vi "多功能示波器.vi"(0 "CH1":bool, 1 "frequency":dbl=10.0 caption="频率" min=0.0 max=1000.0 step=1.0, 2 "频率单位":u16(ring) items=["Hz", "KHz"], 3 "amplitude":dbl=1.0 caption="幅值" min=0.0 max=1000.0 step=1.0 format="%0.2p", 4 "幅值单位":u16(ring) items=["V", "mV"], 5 "phase":dbl caption="相位" format="%.2p", 6 "sampling info":cluster{"Fs":dbl, "#s":dbl}={"Fs"=1000.0, "#s"=1000.0} caption="采样信息" {"Fs" format="%.2p"}) -> ()   [LabVIEW 2020]
uses:
  <vilib>/Analysis/4window.llb/windowTd.ctl
  <vilib>/measure/maspectr.llb/Power Spectrum and PSD Export Mode.ctl
  <vilib>/Analysis/3filter.llb/Filter Structure Type.ctl
  <vilib>/measure/maspectr.llb/FFT Power Spectrum and PSD for N Chan.vi
  <vilib>/measure/macond.llb/FIR Filter for N Chan.vi
  <vilib>/measure/macond.llb/IIR Filter for N Chan.vi
  <vilib>/measure/mascope.llb/Cycle Average and RMS 1 chan.vi
  <vilib>/measure/matone.llb/Extract Single Tone Information 1 Chan.vi
  <vilib>/measure/NI_MABase.lvlib
  <vilib>/measure/NI_MAPro.lvlib
  <vilib>/Analysis/NI_AALPro.lvlib
  <vilib>/Analysis/NI_AALBase.lvlib
panel:
  out "波形参数错误":errorcluster
  in  "选项卡控件 3":enum32{"信号发生器 ", " 滤波模式所用的"}(tab)
  in  "开关":bool
  in  "frequency 2":dbl=10.0 caption="频率" min=0.0 max=1000.0 step=1.0
  in  "频率单位 2":u16(ring) items=["Hz", "KHz"]
  in  "amplitude 2":dbl=1.0 caption="幅值" min=0.0 max=1000.0 step=1.0 format="%0.2p"
  in  "幅值单位  2":u16(ring) items=["V", "mV"]
  in  "phase 2":dbl caption="相位" format="%.2p"
  in  "signal type 2":T1(ring) caption="信号类型"
  in  "CH2":bool
  in  "噪音列表 2":u16(ring) items=["无", "高斯噪音", "均匀白噪音"]
  in  "噪音列表":u16(ring) items=["无", "高斯噪音", "均匀白噪音"]
  in  "signal type":T1(ring) caption="信号类型"
  in  "选项卡控件 2":enum32{"FIR滤波器", " IIR滤波器"}(tab)
  in  "FIR filter specifications":T2={"Topology"=enum."Off", "Type"=enum."Lowpass", "#Taps"=50, "Lower PB"=100.0, "Upper PB"=0.0, "Lower SB"=200.0, "Upper SB"=0.0} caption="FIR滤波器规范" {"Lower SB" format="%0.2p"; "Upper SB" format="%0.2p"; "Lower PB" format="%0.2p"; "Upper PB" format="%0.2p"}
  in  "reset filters":bool caption="重置滤波器"
  in  "filter structure option":T3=10 caption="滤波器结构选项" items=["IIR二阶"=0, "IIR四阶"=1, "自动选择"=10]
  in  "reset filter":bool caption="重置滤波器"
  in  "IIR filter specifications":T4={"Topology"=enum."Butterworth", "Type"=enum."Lowpass", "Order"=1, "Lower Fc"=100.0, "Upper Fc"=200.0, "PB Ripple"=1.0, "SB Attenuation"=60.0} caption="IIR滤波器规范" {"PB Ripple" format="%0.2f"; "SB Attenuation" format="%0.2f"; "Lower Fc" format="%0.2p"; "Upper Fc" format="%0.2p"}
  out "错误输出 3":errorcluster caption="滤波器错误输出"
  out "波形保存错误":errorcluster caption="波形保存错误输出"
  in  "选项卡控件":enum32{"示波器", " 功率频谱测量"}(tab)
  in  "滤波模式":bool
  out "字符串 2":string
  out "字符串":string
  in  "停止波形":bool
  in  "波形回放":bool
  in  "波形保存":bool
  in  "V-mV":bool
  in  "Hz-KHz":bool
  in  "幅值 v/div":dbl(knob) scale=0.0..4.0
  in  "时间 s/div":dbl(knob) scale=0.0..5.0
  out "频率":dbl format="%.2p"
  out "周期平均":dbl format="%.2p"
  out "周期均方根":dbl format="%.2p"
  out "相位":dbl format="%.2p"
  out "幅度":dbl format="%.2p"
  out "周期平均 2":dbl caption="周期平均" format="%.2p"
  out "周期均方根 2":dbl caption="周期均方根" format="%.2p"
  out "相位 2":dbl caption="相位" format="%.2p"
  out "幅度 2":dbl caption="幅度" format="%.2p"
  out "频率 2":dbl caption="频率" format="%.2p"
  out "波形图":waveform(dbl)[](graph)
  out "波形图 2":cluster{"f0":dbl, "df":dbl, "magnitude":dbl[]}[](graph)
  in  "averaging parameters":T5={"averaging mode"=enum."No averaging", "weighting mode"=enum."Exponential", "number of averages"=10} caption="平均参数" {"number of averages" min=1}
  out "averaging done":bool caption="完成平均"
  out "averages completed":dbl caption="已完成平均数"
  in  "restart averaging (F)":bool caption="重新开始平均(F)"
  in  "dB On (F)":bool caption="显示为dB(F)"
  in  "window":T6=1 caption="窗" items=["矩形"=0, "Hanning"=1, "Hamming"=2, "Blackman-Harris"=3, "Exact Blackman"=4, "Blackman"=5, "Flat Top"=6, "4阶Blackman-Harris "=7, "7阶Blackman-Harris"=8, "Low Sidelobe"=9, "Blackman Nuttall"=11, "三角"=30, "Bartlett-Hanning"=31, "Bohman"=32, "Parzen"=33, "Welch"=34, "Kaiser"=60, "Dolph-Chebyshev"=61, "高斯"=62]
  in  "window parameter":dbl=nan caption="窗参数"
  in  "export mode":T7 caption="导出模式" items=["功率谱", "功率谱密度"]
  out "error out 2":errorcluster caption="波形保存错误"
  out "error out":errorcluster caption="信号发生错误显示"
  # "信号发生器"
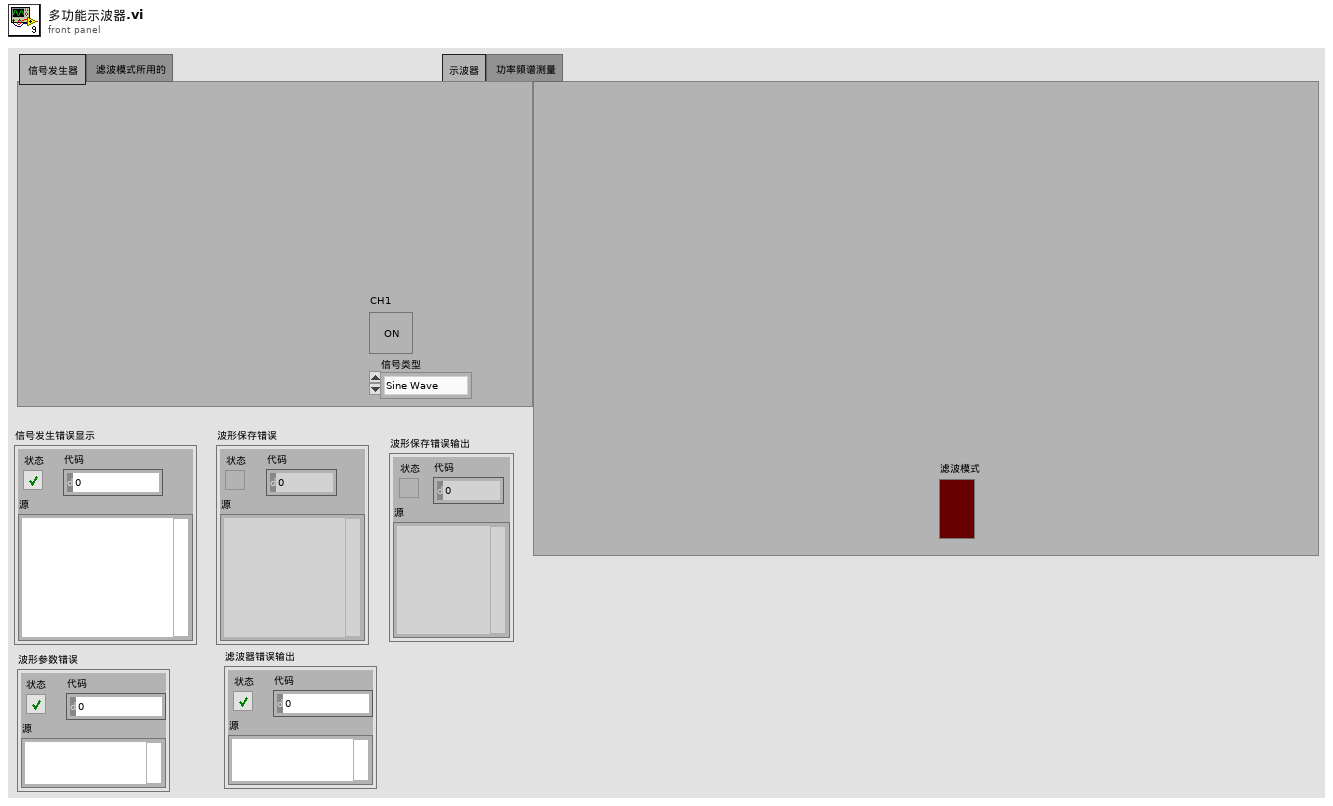
[diagram p1: front panel]
types:
  T1 = enum16{"Sine Wave", "Triangle Wave", "Square Wave", "Sawtooth Wave"}
  T2 = cluster{"Topology":enum16{"Off", "FIR by Specification", "Equi-ripple FIR", "Windowed FIR"}, "Type":enum16{"Lowpass", "Highpass", "Bandpass", "Bandstop"}, "#Taps":i32, "Lower PB":dbl, "Upper PB":dbl, "Lower SB":dbl, "Upper SB":dbl}
  T3 = typedef "NI_AALBase.lvlib/Filter Structure Type.ctl" = u16
  T4 = cluster{"Topology":enum16{"Off", "Butterworth", "Chebyshev", "Inverse Chebyshev", "Elliptic", "Bessel"}, "Type":enum16{"Lowpass", "Highpass", "Bandpass", "Bandstop"}, "Order":i32, "Lower Fc":dbl, "Upper Fc":dbl, "PB Ripple":dbl, "SB Attenuation":dbl}
  T5 = cluster{"averaging mode":enum16{"No averaging", "Vector averaging", "RMS averaging", "Peak hold"}, "weighting mode":enum16{"Linear", "Exponential"}, "number of averages":u32}
  T6 = typedef "NI_AALPro.lvlib/windowTd.ctl" = u32
  T7 = typedef "NI_MAPro.lvlib/Power Spectrum and PSD Export Mode.ctl" = u16
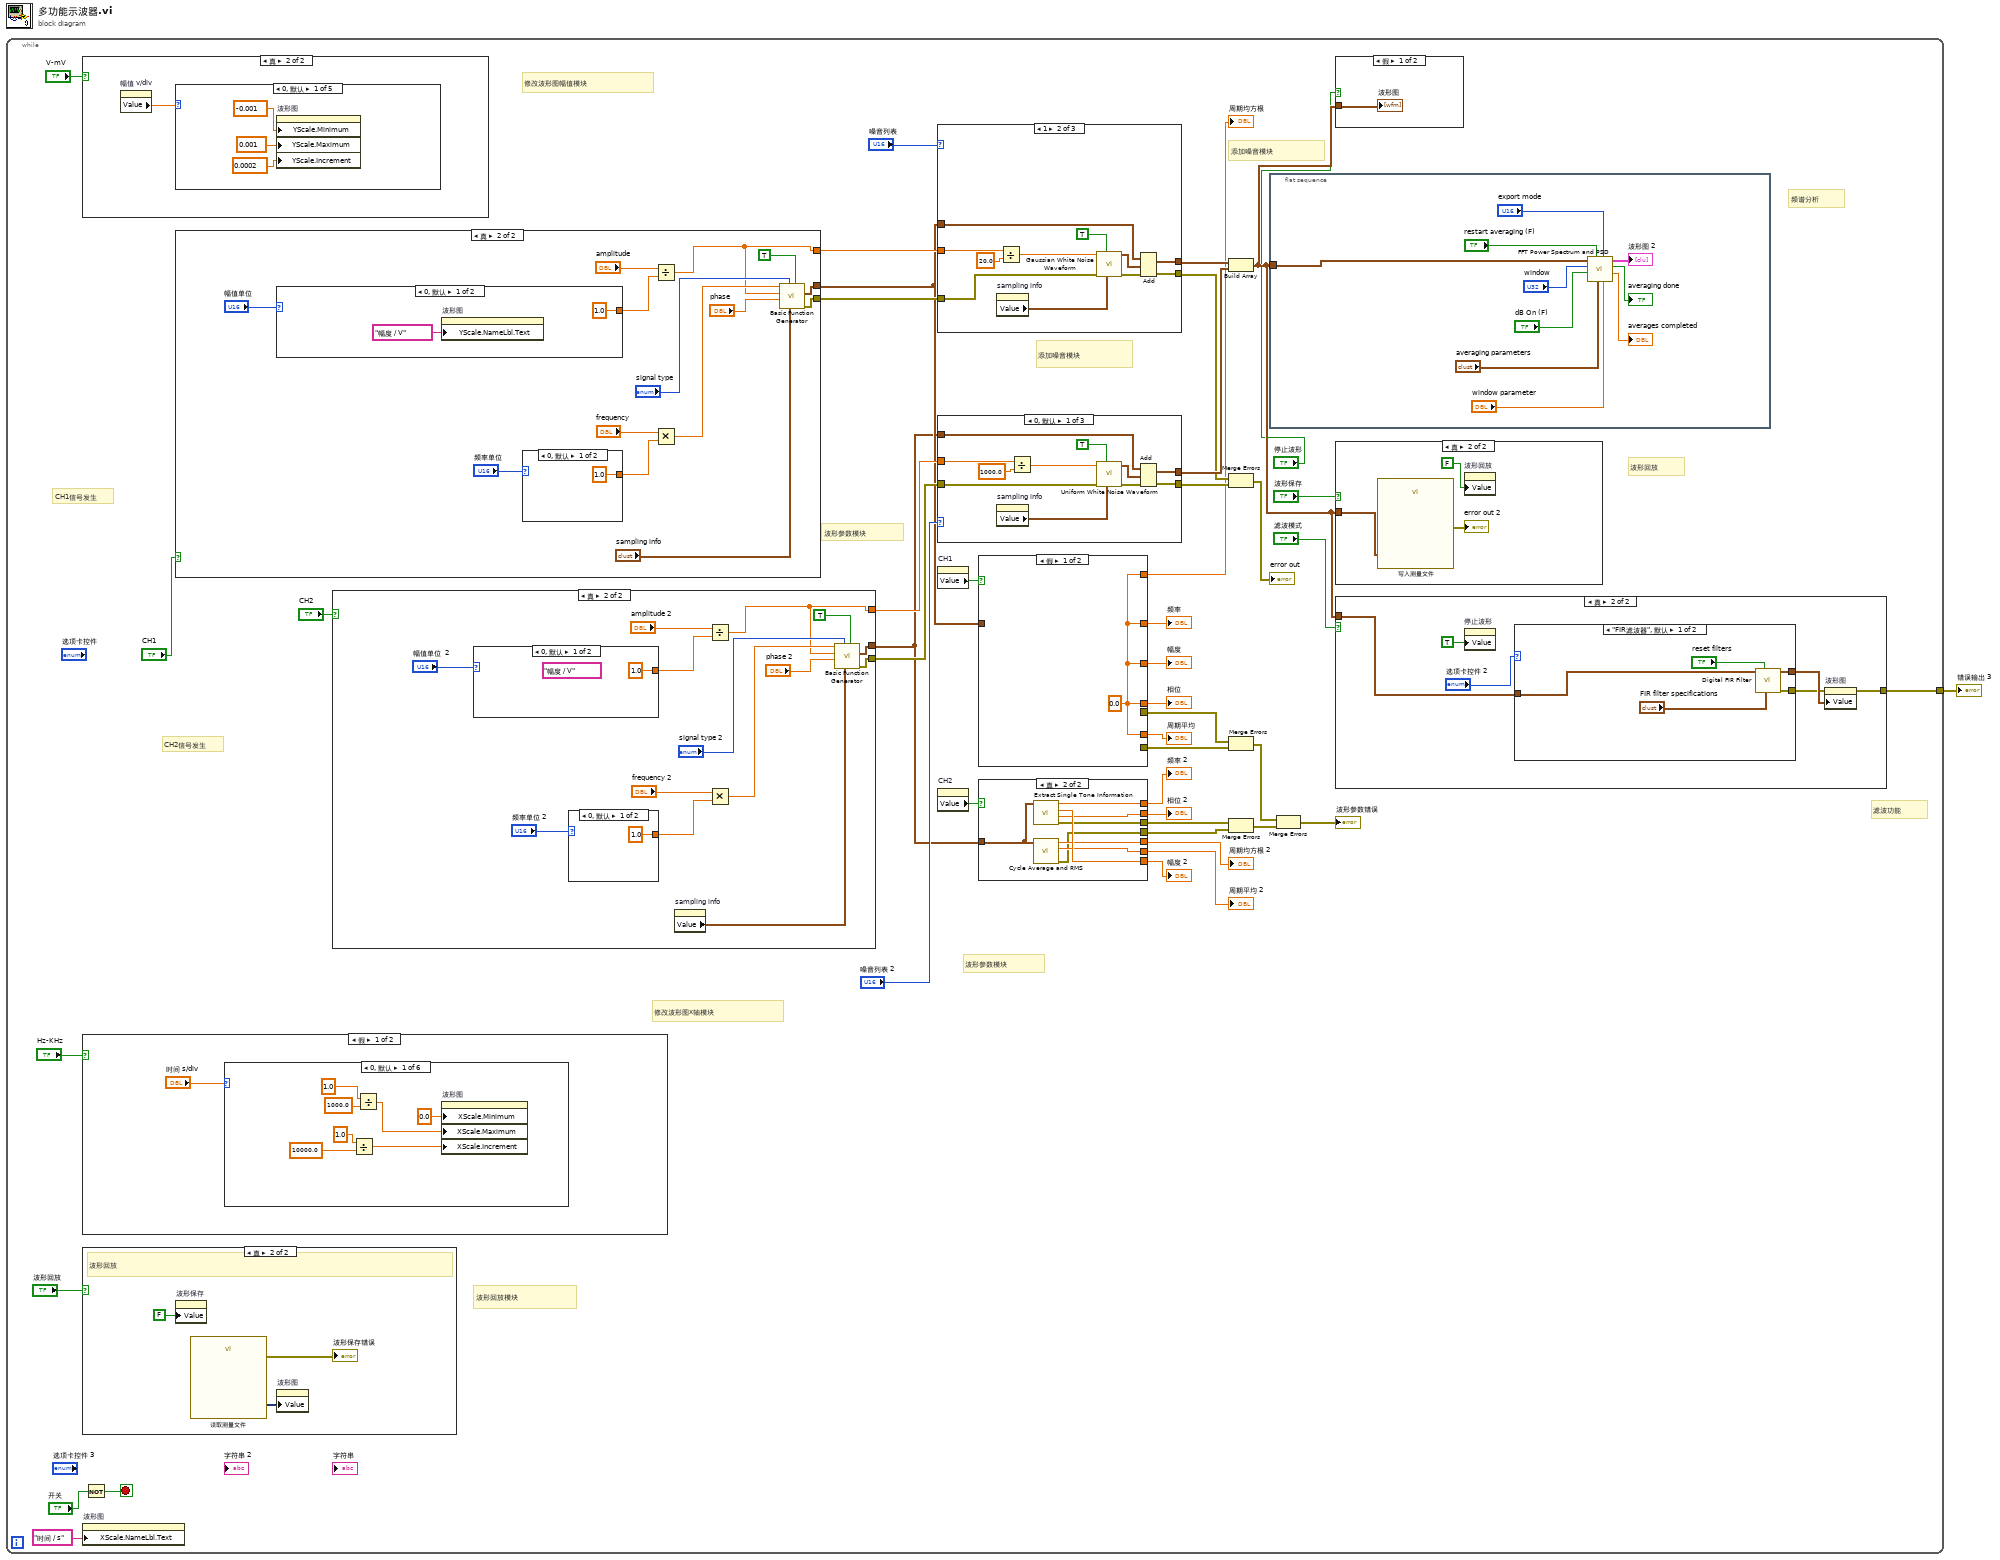
[diagram p0: block diagram]
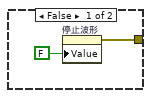
[diagram p2: hidden frame]
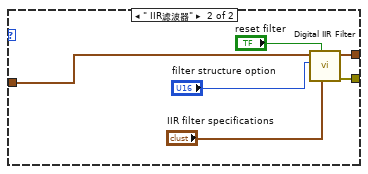
[diagram p3: hidden frame]
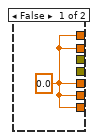
[diagram p4: hidden frame]
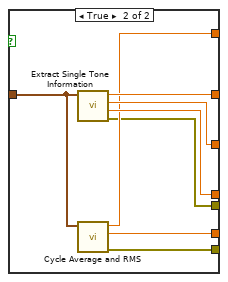
[diagram p5: hidden frame]
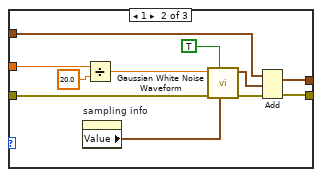
[diagram p9: hidden frame]
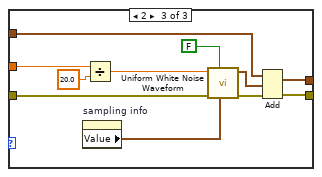
[diagram p10: hidden frame]
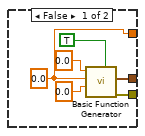
[diagram p11: hidden frame]
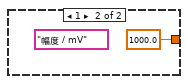
[diagram p12: hidden frame]
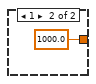
[diagram p13: hidden frame]
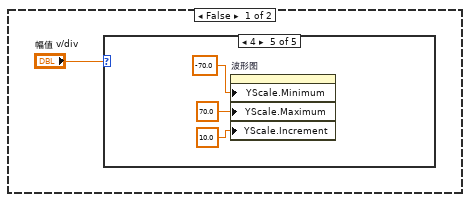
[diagram p14: hidden frame]
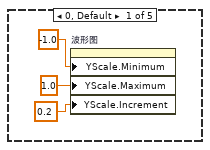
[diagram p15: hidden frame]
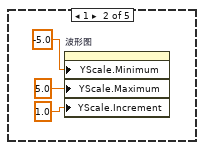
[diagram p16: hidden frame]
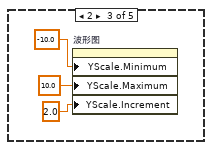
[diagram p17: hidden frame]
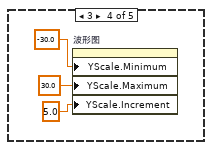
[diagram p18: hidden frame]
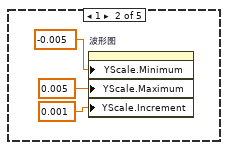
[diagram p19: hidden frame]
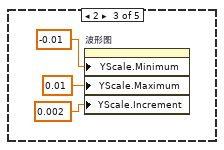
[diagram p20: hidden frame]
diagram:
  n1 = while {
    tunnel: [w5] -> w1
    stop <- w44 stop-if-true
    # "滤波功能"
    # "频谱分析"
    # "波形回放"
    # "波形参数模块"
    # "波形参数模块"
    # "添加噪音模块"
    # "添加噪音模块"
    # "CH2信号发生"
    # "CH1信号发生"
    # "修改波形图x轴模块"
    # "修改波形图幅值模块"
    # "波形回放模块"
    n2 = case shown="真" "V-mV" {
      frame False {
        n3 = case shown="4" "幅值 v/div" {
          frame 0, Default {
            n4 = property on="波形图" class="WFGraph (严格)"("YScale.Minimum"=-1.0 ("Y标尺.范围:最小值"), "YScale.Maximum"=1.0 ("Y标尺.范围:最大值"), "YScale.Increment"=0.2 ("Y标尺.范围:增量")) -> ()  [unwired: 2 in, 2 out]
          }
          frame 1 {
            n5 = property on="波形图" class="WFGraph (严格)"("YScale.Minimum"=-5.0 ("Y标尺.范围:最小值"), "YScale.Maximum"=5.0 ("Y标尺.范围:最大值"), "YScale.Increment"=1.0 ("Y标尺.范围:增量")) -> ()  [unwired: 2 in, 2 out]
          }
          frame 2 {
            n6 = property on="波形图" class="WFGraph (严格)"("YScale.Minimum"=-10.0 ("Y标尺.范围:最小值"), "YScale.Maximum"=10.0 ("Y标尺.范围:最大值"), "YScale.Increment"=2.0 ("Y标尺.范围:增量")) -> ()  [unwired: 2 in, 2 out]
          }
          frame 3 {
            n7 = property on="波形图" class="WFGraph (严格)"("YScale.Minimum"=-30.0 ("Y标尺.范围:最小值"), "YScale.Maximum"=30.0 ("Y标尺.范围:最大值"), "YScale.Increment"=5.0 ("Y标尺.范围:增量")) -> ()  [unwired: 2 in, 2 out]
          }
          frame 4 {
            n8 = property on="波形图" class="WFGraph (严格)"("YScale.Minimum"=-70.0 ("Y标尺.范围:最小值"), "YScale.Maximum"=70.0 ("Y标尺.范围:最大值"), "YScale.Increment"=10.0 ("Y标尺.范围:增量")) -> ()  [unwired: 2 in, 2 out]
          }
        }
      }
      frame True {
        n9 = property on="幅值 v/div" class="Knob (严格)"() -> ("Value"=w174:dbl)  [unwired: 2 in, 2 out]
        n10 = case shown="0, 默认" w174 {
          frame 0, Default {
            n11 = property on="波形图" class="WFGraph (严格)"("YScale.Minimum"=-0.001 ("Y标尺.范围:最小值"), "YScale.Maximum"=0.001 ("Y标尺.范围:最大值"), "YScale.Increment"=0.0002 ("Y标尺.范围:增量")) -> ()  [unwired: 2 in, 2 out]
          }
          frame 1 {
            n12 = property on="波形图" class="WFGraph (严格)"("YScale.Minimum"=-0.005 ("Y标尺.范围:最小值"), "YScale.Maximum"=0.005 ("Y标尺.范围:最大值"), "YScale.Increment"=0.001 ("Y标尺.范围:增量")) -> ()  [unwired: 2 in, 2 out]
          }
          frame 2 {
            n13 = property on="波形图" class="WFGraph (严格)"("YScale.Minimum"=-0.01 ("Y标尺.范围:最小值"), "YScale.Maximum"=0.01 ("Y标尺.范围:最大值"), "YScale.Increment"=0.002 ("Y标尺.范围:增量")) -> ()  [unwired: 2 in, 2 out]
          }
          frame 3 {
            n14 = property on="波形图" class="WFGraph (严格)"("YScale.Minimum"=-0.03 ("Y标尺.范围:最小值"), "YScale.Maximum"=0.03 ("Y标尺.范围:最大值"), "YScale.Increment"=0.005 ("Y标尺.范围:增量")) -> ()  [unwired: 2 in, 2 out]
          }
          frame 4 {
            n15 = property on="波形图" class="WFGraph (严格)"("YScale.Minimum"=-0.07 ("Y标尺.范围:最小值"), "YScale.Maximum"=0.07 ("Y标尺.范围:最大值"), "YScale.Increment"=0.01 ("Y标尺.范围:增量")) -> ()  [unwired: 2 in, 2 out]
          }
        }
      }
    }
    n16 = case shown="假" "Hz-KHz" {
      frame False {
        n17 = case shown="0, 默认" "时间 s/div" {
          frame 0, Default {
            n18 = Divide(x=1.0, y=10000.0) -> (x/y=w191:dbl)
            n19 = Divide(x=1.0, y=1000.0) -> (x/y=w194:dbl)
            n20 = property on="波形图" class="WFGraph (严格)"("XScale.Minimum"=0.0 ("X标尺.范围:最小值"), "XScale.Maximum"=w194, "XScale.Increment"=w191) -> ()  [unwired: 2 in, 2 out]
          }
          frame 1 {
            n21 = Divide(x=1.0, y=1000.0) -> (x/y=w198:dbl)
            n22 = Divide(x=1.0, y=100.0) -> (x/y=w201:dbl)
            n23 = property on="波形图" class="WFGraph (严格)"("XScale.Minimum"=0.0 ("X标尺.范围:最小值"), "XScale.Maximum"=w201, "XScale.Increment"=w198) -> ()  [unwired: 2 in, 2 out]
          }
          frame 2 {
            n24 = Divide(x=5.0, y=1000.0) -> (x/y=w205:dbl)
            n25 = Divide(x=5.0, y=100.0) -> (x/y=w208:dbl)
            n26 = property on="波形图" class="WFGraph (严格)"("XScale.Minimum"=0.0 ("X标尺.范围:最小值"), "XScale.Maximum"=w208, "XScale.Increment"=w205) -> ()  [unwired: 2 in, 2 out]
          }
          frame 3 {
            n27 = Divide(x=1.0, y=10.0) -> (x/y=w215:dbl)
            n28 = Divide(x=1.0, y=100.0) -> (x/y=w212:dbl)
            n29 = property on="波形图" class="WFGraph (严格)"("XScale.Minimum"=0.0 ("X标尺.范围:最小值"), "XScale.Maximum"=w215, "XScale.Increment"=w212) -> ()  [unwired: 2 in, 2 out]
          }
          frame 4 {
            n30 = Divide(x=15.0, y=1000.0) -> (x/y=w219:dbl)
            n31 = Divide(x=15.0, y=100.0) -> (x/y=w222:dbl)
            n32 = property on="波形图" class="WFGraph (严格)"("XScale.Minimum"=0.0 ("X标尺.范围:最小值"), "XScale.Maximum"=w222, "XScale.Increment"=w219) -> ()  [unwired: 2 in, 2 out]
          }
          frame 5 {
            n33 = Divide(x=2.0, y=10.0) -> (x/y=w232:dbl)
            n34 = Divide(x=2.0, y=100.0) -> (x/y=w231:dbl)
            n35 = property on="波形图" class="WFGraph (严格)"("XScale.Minimum"=0.0 ("X标尺.范围:最小值"), "XScale.Maximum"=w232, "XScale.Increment"=w231) -> ()  [unwired: 2 in, 2 out]
          }
        }
      }
      frame True {
        n36 = property on="时间 s/div" class="Knob (严格)"() -> ("Value"=w233:dbl)  [unwired: 2 in, 2 out]
        n37 = case shown="4" w233 {
          frame 0, Default {
            n38 = Divide(x=1.0, y=1000000.0) -> (x/y=w237:dbl)
            n39 = Divide(x=1.0, y=10000000.0) -> (x/y=w234:dbl)
            n40 = property on="波形图" class="WFGraph (严格)"("XScale.Minimum"=0.0 ("X标尺.范围:最小值"), "XScale.Maximum"=w237, "XScale.Increment"=w234) -> ()  [unwired: 2 in, 2 out]
          }
          frame 1 {
            n41 = Divide(x=1.0, y=100000.0) -> (x/y=w244:dbl)
            n42 = Divide(x=1.0, y=1000000.0) -> (x/y=w241:dbl)
            n43 = property on="波形图" class="WFGraph (严格)"("XScale.Minimum"=0.0 ("X标尺.范围:最小值"), "XScale.Maximum"=w244, "XScale.Increment"=w241) -> ()  [unwired: 2 in, 2 out]
          }
          frame 2 {
            n44 = Divide(x=5.0, y=100000.0) -> (x/y=w251:dbl)
            n45 = Divide(x=5.0, y=1000000.0) -> (x/y=w248:dbl)
            n46 = property on="波形图" class="WFGraph (严格)"("XScale.Minimum"=0.0 ("X标尺.范围:最小值"), "XScale.Maximum"=w251, "XScale.Increment"=w248) -> ()  [unwired: 2 in, 2 out]
          }
          frame 3 {
            n47 = Divide(x=1.0, y=10000.0) -> (x/y=w258:dbl)
            n48 = Divide(x=1.0, y=100000.0) -> (x/y=w255:dbl)
            n49 = property on="波形图" class="WFGraph (严格)"("XScale.Minimum"=0.0 ("X标尺.范围:最小值"), "XScale.Maximum"=w258, "XScale.Increment"=w255) -> ()  [unwired: 2 in, 2 out]
          }
          frame 4 {
            n50 = Divide(x=15.0, y=100000.0) -> (x/y=w265:dbl)
            n51 = Divide(x=15.0, y=1000000.0) -> (x/y=w262:dbl)
            n52 = property on="波形图" class="WFGraph (严格)"("XScale.Minimum"=0.0 ("X标尺.范围:最小值"), "XScale.Maximum"=w265, "XScale.Increment"=w262) -> ()  [unwired: 2 in, 2 out]
          }
          frame 5 {
            n53 = Divide(x=2.0, y=10000.0) -> (x/y=w275:dbl)
            n54 = Divide(x=2.0, y=100000.0) -> (x/y=w274:dbl)
            n55 = property on="波形图" class="WFGraph (严格)"("XScale.Minimum"=0.0 ("X标尺.范围:最小值"), "XScale.Maximum"=w275, "XScale.Increment"=w274) -> ()  [unwired: 2 in, 2 out]
          }
        }
      }
    }
    n56 = case shown="真" "波形回放" {
      frame False {
      }
      frame True {
        # "波形回放"
        n57 = property on="波形保存" class="Bool (严格)"("Value"=FALSE ("波形保存")) -> ()  [unwired: 2 in, 2 out]
        n58 = call "读取测量文件"() -> ("error out"=→"波形保存错误":errorcluster, "Signals"=w97:dynamicdata)  [unwired: 6 in, 4 out]
        n59 = property on="波形图" class="WFGraph (严格)"("Value"=w97) -> ()  [unwired: 2 in, 2 out]
      }
    }
    n60 = property on="波形图" class="WFGraph (严格)"("XScale.NameLbl.Text"="时间 / s" ("X标尺.名称标签.文本")) -> ()  [unwired: 2 in, 2 out]
    n61 = Not(x="开关") -> (.not. x?=w44:bool)
    n62 = case shown="真" "CH1" {
      tunnel: [w312 w318] -> w26
      tunnel: [w311 w317] -> w42
      tunnel: [w310 w316] -> w41
      frame False {
        w310 = 0.0 ("amplitude")
        n63 = property on="sampling info" class="Clust (严格)"() -> ("Value"=w309:cluster{"Fs":dbl, "#s":dbl})  [unwired: 2 in, 2 out]
        n64 = call <vilib>:"Basic Function Generator.vi"("reset signal"=TRUE, "sampling info"=w309, "phase"=0.0, "amplitude"=w310, "frequency"=0.0) -> ("error out"=w311:errorcluster, "signal out"=w312:waveform(dbl))  [unwired: 4 in, 1 out]
      }
      frame True {
        n65 = case shown="0, 默认" "幅值单位" {
          tunnel: [1.0 1000.0] -> w322
          frame 0, Default {
            n66 = property on="波形图" class="WFGraph (严格)"("YScale.NameLbl.Text"="幅度 / V") -> ()  [unwired: 2 in, 2 out]
          }
          frame 1 {
            n67 = property on="波形图" class="WFGraph (严格)"("YScale.NameLbl.Text"="幅度 / mV") -> ()  [unwired: 2 in, 2 out]
          }
        }
        n68 = case shown="0, 默认" "频率单位" {
          tunnel: [1.0 1000.0] -> w327
          frame 0, Default {
          }
          frame 1 {
          }
        }
        n69 = Divide(x="amplitude", y=w322) -> (x/y=w316:dbl)
        n70 = Multiply(x="frequency", y=w327) -> (x*y=w326:dbl)
        n71 = call <vilib>:"Basic Function Generator.vi"("reset signal"=TRUE, "sampling info"="sampling info", "signal type"="signal type", "phase"="phase", "amplitude"=w316, "frequency"=w326) -> ("error out"=w317:errorcluster, "signal out"=w318:waveform(dbl))  [unwired: 3 in, 1 out]
      }
    }
    n72 = case shown="真" "CH2" {
      tunnel: [w136 w143] -> w10
      tunnel: [w135 w142] -> w36
      tunnel: [w134 w141] -> w37
      frame False {
        w134 = 0.0 ("amplitude")
        n73 = call <vilib>:"Basic Function Generator.vi"("reset signal"=TRUE, "phase"=0.0, "amplitude"=w134, "frequency"=0.0) -> ("error out"=w135:errorcluster, "signal out"=w136:waveform(dbl))  [unwired: 5 in, 1 out]
      }
      frame True {
        n74 = case shown="0, 默认" "幅值单位  2" {
          tunnel: [1.0 1000.0] -> w147
          frame 0, Default {
            (unwired) "幅度 / V"
          }
          frame 1 {
            (unwired) "幅度 / mV"
          }
        }
        n75 = case shown="0, 默认" "频率单位 2" {
          tunnel: [1.0 1000.0] -> w151
          frame 0, Default {
          }
          frame 1 {
          }
        }
        n76 = property on="sampling info" class="Clust (严格)"() -> ("Value"=w140:cluster{"Fs":dbl, "#s":dbl})  [unwired: 2 in, 2 out]
        n77 = Divide(x="amplitude 2", y=w147) -> (x/y=w141:dbl)
        n78 = Multiply(x="frequency 2", y=w151) -> (x*y=w150:dbl)
        n79 = call <vilib>:"Basic Function Generator.vi"("reset signal"=TRUE, "sampling info"=w140, "signal type"="signal type 2", "phase"="phase 2", "amplitude"=w141, "frequency"=w150) -> ("error out"=w142:errorcluster, "signal out"=w143:waveform(dbl))  [unwired: 3 in, 1 out]
      }
    }
    n80 = case shown="1" "噪音列表" {
      tunnel: w26 -> [w281 w292 w304]
      tunnel: w42 -> [w278 w290 w301]
      tunnel: w41 -> [w285 w296 w307]
      tunnel: [w280 w291 w303] -> w32
      tunnel: [w277 w288 w299] -> w30
      frame 0, Default {
        n81 = property on="sampling info" class="Clust (严格)"() -> ("Value"=w276:cluster{"Fs":dbl, "#s":dbl})  [unwired: 2 in, 2 out]
        n82 = Divide(x=w285, y=1000.0) -> (x/y=w283:dbl)
        n83 = call <vilib>:"Uniform White Noise Waveform.vi"("sampling info"=w276, "reset signal"=TRUE, "error in (no error)"=w278, "amplitude"=w283) -> ("error out"=w279:errorcluster, "signal out"=w282:waveform(dbl))  [unwired: 6 in]
        n84 = Add(1:w282, 2:w281, 4:w279) -> (0:w280:waveform(dbl), 3:w277:errorcluster)
      }
      frame 1 {
        n85 = property on="sampling info" class="Clust (严格)"() -> ("Value"=w287:cluster{"Fs":dbl, "#s":dbl})  [unwired: 2 in, 2 out]
        n86 = Divide(x=w296, y=20.0) -> (x/y=w294:dbl)
        n87 = call <vilib>:"Gaussian White Noise Waveform.vi"("sampling info"=w287, "reset signal"=TRUE, "error in (no error)"=w290, "standard deviation"=w294) -> ("error out"=w289:errorcluster, "signal out"=w293:waveform(dbl))  [unwired: 6 in]
        n88 = Add(1:w293, 2:w292, 4:w289) -> (0:w291:waveform(dbl), 3:w288:errorcluster)
      }
      frame 2 {
        n89 = property on="sampling info" class="Clust (严格)"() -> ("Value"=w298:cluster{"Fs":dbl, "#s":dbl})  [unwired: 2 in, 2 out]
        n90 = Divide(x=w307, y=20.0) -> (x/y=w305:dbl)
        n91 = call <vilib>:"Uniform White Noise Waveform.vi"("sampling info"=w298, "reset signal"=FALSE, "error in (no error)"=w301, "amplitude"=w305) -> ("error out"=w300:errorcluster, "signal out"=w302:waveform(dbl))  [unwired: 6 in]
        n92 = Add(1:w302, 2:w304, 4:w300) -> (0:w303:waveform(dbl), 3:w299:errorcluster)
      }
    }
    n93 = case shown="0, 默认" "噪音列表 2" {
      tunnel: w10 -> [w106 w117 w129]
      tunnel: w36 -> [w103 w115 w126]
      tunnel: w37 -> [w110 w121 w132]
      tunnel: [w105 w116 w128] -> w33
      tunnel: [w102 w113 w124] -> w31
      frame 0, Default {
        n94 = property on="sampling info" class="Clust (严格)"() -> ("Value"=w101:cluster{"Fs":dbl, "#s":dbl})  [unwired: 2 in, 2 out]
        n95 = Divide(x=w110, y=1000.0) -> (x/y=w108:dbl)
        n96 = call <vilib>:"Uniform White Noise Waveform.vi"("sampling info"=w101, "reset signal"=TRUE, "error in (no error)"=w103, "amplitude"=w108) -> ("error out"=w104:errorcluster, "signal out"=w107:waveform(dbl))  [unwired: 6 in]
        n97 = Add(1:w107, 2:w106, 4:w104) -> (0:w105:waveform(dbl), 3:w102:errorcluster)
      }
      frame 1 {
        n98 = property on="sampling info" class="Clust (严格)"() -> ("Value"=w112:cluster{"Fs":dbl, "#s":dbl})  [unwired: 2 in, 2 out]
        n99 = Divide(x=w121, y=20.0) -> (x/y=w119:dbl)
        n100 = call <vilib>:"Gaussian White Noise Waveform.vi"("sampling info"=w112, "reset signal"=TRUE, "error in (no error)"=w115, "standard deviation"=w119) -> ("error out"=w114:errorcluster, "signal out"=w118:waveform(dbl))  [unwired: 6 in]
        n101 = Add(1:w118, 2:w117, 4:w114) -> (0:w116:waveform(dbl), 3:w113:errorcluster)
      }
      frame 2 {
        n102 = property on="sampling info" class="Clust (严格)"() -> ("Value"=w123:cluster{"Fs":dbl, "#s":dbl})  [unwired: 2 in, 2 out]
        n103 = Divide(x=w132, y=20.0) -> (x/y=w130:dbl)
        n104 = call <vilib>:"Uniform White Noise Waveform.vi"("sampling info"=w123, "reset signal"=FALSE, "error in (no error)"=w126, "amplitude"=w130) -> ("error out"=w125:errorcluster, "signal out"=w127:waveform(dbl))  [unwired: 6 in]
        n105 = Add(1:w127, 2:w129, 4:w125) -> (0:w128:waveform(dbl), 3:w124:errorcluster)
      }
    }
    n106 = property on="CH1" class="Bool (严格)"() -> ("Value"=w25:bool)  [unwired: 2 in, 2 out]
    n107 = property on="CH2" class="Bool (严格)"() -> ("Value"=w9:bool)  [unwired: 2 in, 2 out]
    n108 = case shown="假" w25 {
      tunnel: w26 -> [_ w93]
      tunnel: [w85 w92] -> w24
      tunnel: [w85 w91] -> w23
      tunnel: [w85 w90] -> w22
      tunnel: [w85 w89] -> w21
      tunnel: [w85 w88] -> w20
      tunnel: [_ w87] -> w19
      tunnel: [_ w86] -> w18
      frame False {
        w85 = 0.0
      }
      frame True {
        n109 = call-poly <vilib>:"Extract Single Tone Information.vi"("time signal in"=w93) -> ("error out"=w87:errorcluster, "detected phase (deg)"=w90:dbl, "detected amplitude"=w91:dbl, "detected frequency"=w92:dbl)  [unwired: 5 in, 2 out]
        n110 = call-poly <vilib>:"Cycle Average and RMS.vi"("signal in"=w93) -> ("error out"=w86:errorcluster, "cycle RMS"=w88:dbl, "cycle average"=w89:dbl)  [unwired: 7 in, 1 out]
      }
    }
    "频率" <- w24
    "幅度" <- w23
    "相位" <- w22
    "周期均方根" <- w21
    "周期平均" <- w20
    n111 = case shown="真" w9 {
      tunnel: w10 -> [_ w84]
      tunnel: [w76 w83] -> w11
      tunnel: [w76 w82] -> w12
      tunnel: [w76 w81] -> w13
      tunnel: [w76 w80] -> w14
      tunnel: [w76 w79] -> w15
      tunnel: [_ w78] -> w16
      tunnel: [_ w77] -> w17
      frame False {
        w76 = 0.0
      }
      frame True {
        n112 = call-poly <vilib>:"Extract Single Tone Information.vi"("time signal in"=w84) -> ("error out"=w78:errorcluster, "detected phase (deg)"=w81:dbl, "detected amplitude"=w82:dbl, "detected frequency"=w83:dbl)  [unwired: 5 in, 2 out]
        n113 = call-poly <vilib>:"Cycle Average and RMS.vi"("signal in"=w84) -> ("error out"=w77:errorcluster, "cycle RMS"=w79:dbl, "cycle average"=w80:dbl)  [unwired: 7 in, 1 out]
      }
    }
    "频率 2" <- w11
    "幅度 2" <- w12
    "相位 2" <- w13
    "周期均方根 2" <- w14
    "周期平均 2" <- w15
    n114 = Build Array(w32, w33) -> (w7:waveform(dbl)[])
    n115 = Merge Errors(w30, w31) -> (→"error out":errorcluster)
    n116 = Merge Errors(w19, w18) -> (w4:errorcluster)
    n117 = Merge Errors(w16, w17) -> (w3:errorcluster)
    n118 = flat-sequence {
      tunnel: w7 -> [w75]
      frame #0 {
        n119 = call-poly <vilib>:"FFT Power Spectrum and PSD.vi"("window parameter"="window parameter", "export mode"="export mode", "averaging parameters"="averaging parameters", "restart averaging (F)"="restart averaging (F)", "dB On (F)"="dB On (F)", "window"="window", "time signals"=w75) -> ("averages completed"=→"averages completed":dbl, "averaging done"=→"averaging done":bool, "Power Spectrum / PSD"=→"波形图 2":cluster{"f0":dbl, "df":dbl, "magnitude":dbl[]}[])  [unwired: 1 in, 1 out]
      }
    }
    n120 = Merge Errors(w4, w3) -> (→"波形参数错误":errorcluster)
    n121 = case shown="假" "停止波形" {
      tunnel: w7 -> [w94 _]
      frame False {
        "波形图" <- w94
      }
      frame True {
      }
    }
    n122 = case shown="真" "波形保存" {
      tunnel: w7 -> [_ w100]
      frame False {
      }
      frame True {
        n123 = call "写入测量文件"("Signals"=w100) -> ("error out"=→"error out 2":errorcluster)  [unwired: 16 in, 2 out]
        n124 = property on="波形回放" class="Bool (严格)"("Value"=FALSE ("波形回放")) -> ()  [unwired: 2 in, 2 out]
      }
    }
    n125 = case shown="真" "滤波模式" {
      tunnel: w7 -> [_ w53]
      tunnel: [w47 w49] -> w5
      frame False {
        n126 = property on="停止波形" class="Bool (严格)"("Value"=FALSE ("波形保存")) -> (error out=w47:errorcluster)  [unwired: 2 in, 1 out]
      }
      frame True {
        n127 = property on="停止波形" class="Bool (严格)"("Value"=TRUE ("停止波形")) -> ()  [unwired: 2 in, 2 out]
        n128 = case shown="\"FIR滤波器\", 默认" "选项卡控件 2" {
          tunnel: w53 -> [w59 w65]
          tunnel: [w57 w61] -> w51
          tunnel: [w55 w60] -> w50
          frame "FIR滤波器", Default {
            n129 = call-poly <vilib>:"Digital FIR Filter.vi"("FIR filter specifications"="FIR filter specifications", "reset filters"="reset filters", "signal(s) in"=w59) -> ("error out"=w55:errorcluster, "signal(s) out"=w57:waveform(dbl)[])  [unwired: 6 in, 1 out]
          }
          frame " IIR滤波器" {
            n130 = call-poly <vilib>:"Digital IIR Filter.vi"("IIR filter specifications"="IIR filter specifications", "reset filters"="reset filter", "filter structure option"="filter structure option", "signal(s) in"=w65) -> ("error out"=w60:errorcluster, "signal(s) out"=w61:waveform(dbl)[])  [unwired: 5 in, 1 out]
          }
        }
        n131 = property on="波形图" class="WFGraph (严格)"(error in=w50, "Value"=w51) -> (error out=w49:errorcluster)  [unwired: 1 in, 1 out]
      }
    }
  }
  "错误输出 3" <- w1
